vi "Get_OutputSignal.vi"(8 "error in":errorcluster, 11 "camera handle in":u64) -> (0 "error out":errorcluster, 1 "PicamOutputSignal_":T1=1 items=["NotReadingOut"=1, "ShutterOpen"=2, "Busy"=3, "AlwaysLow"=4, "AlwaysHigh"=5, "Acquiring"=6, "ShiftingUnderMask"=7, "Exposing"=8, "EffectivelyExposing"=9, "ReadingOut"=10, "WaitingForTrigger"=11, "InternalTriggerT0"=12, "Gate"=13, "AuxOutput"=14, "EffectivelyExposingAlternation"=15], 3 "camera handle out":u64)   [LabVIEW 2019, in "PICam.lvlib"]
doc: "PicamAdcAnalogGain is the set of electronic gain settings for pixel digitization.\n\nPicamAdcAnalogGain_Low Small amplification.\nPicamAdcAnalogGain_Medium Average amplification.\nPicamAdcAnalogGain_High Large amplification.\n\nRefer to the user manual for the specific\ncamera being used for complete information."
uses:
  PICam.lvlib
  Ctrls/PicamOutputSignal.ctl
  Picam64.dll   
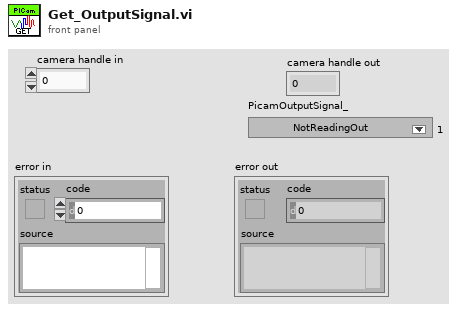
[diagram p1: front panel]
types:
  T1 = typedef "PICam.lvlib/PicamOutputSignal.ctl" = u32
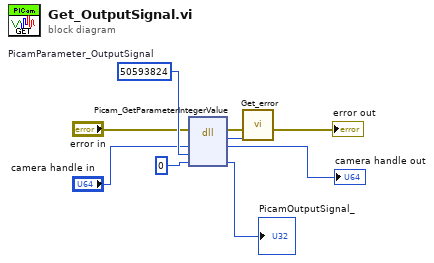
[diagram p0: block diagram]
diagram:
  w5 = u32 50593824  # PicamParameter_OutputSignal
  n1 = dll-call lib="Picam32.dll" fn="Picam_GetParameterIntegerValue"(error in="error in", "camera"="camera handle in", "PicamParameter"=w5, "OutputSignal"=u32 0 ("AdcAnalogGain")) -> (error out=w9:errorcluster, "return type"=w8:i32, "camera"=→"camera handle out":u64, "OutputSignal"=→"PicamOutputSignal_":u32)  [unwired: 3 in, 1 out]
  n2 = call "Get_error.vi"("PICam_Error"=w8, "error in (no error)"=w9) -> ("error out"=→"error out":errorcluster)  [unwired: 9 in]
